vi "Core Actor - Close User Events.vi"(8 "error in (no error)":errorcluster, 11 "Parent_Class in":refnum<class "Message_Distributor_Class.lvclass">) -> (0 "error out":errorcluster, 3 "Parent_Class out":refnum<class "Message_Distributor_Class.lvclass">)   [LabVIEW 2023, in "Actor_Message_Distributor.lvlib" / "Message_Distributor_Class.lvclass"]
uses:
  Message_Distributor_Class.lvclass
  Usr Ev/Distributor - Ctrl - Action.ctl
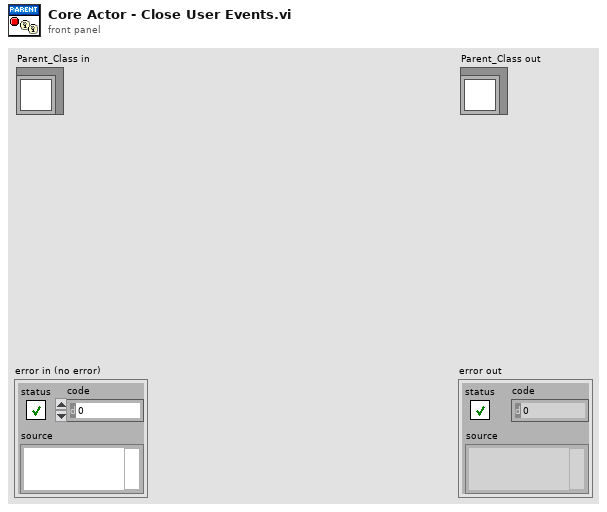
[diagram p1: front panel]
types:
  T1 = typedef "Actor_Message_Distributor.lvlib/Message_Distributor_Class.lvclass/Distributor - Ctrl - Action.ctl" = enum16{"Reg Ev", "Get Refs", "Close Ev", "Populate Enum with Events"}
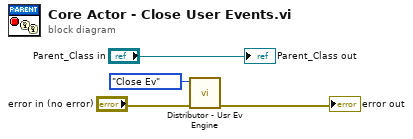
[diagram p0: block diagram]
diagram:
  n1 = call "Distributor - Usr Ev Engine.vi"("error in (no error)"="error in (no error)", "Action"=Distributor_-_Ctrl_-_Action."Close Ev") -> ("error out"=→"error out":errorcluster)  [unwired: 6 in, 3 out]
  "Parent_Class out" <- "Parent_Class in"
